vi "ISX3_Get_All_ISX3.vi"() -> (1 "A list of FT_Handel where an ISX-3 is connected to.\nThis handle must be used for further interaction \nwith the USB interface.":u32[](array[numeric]) format="%x")   [LabVIEW 2012, in "Sciospec ISX3 Impedance Analyzer.lvlib"]
uses:
  Sciospec ISX3 Impedance Analyzer.lvlib
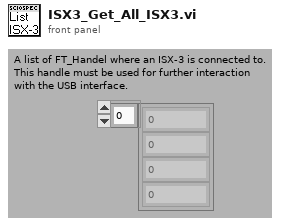
[diagram p1: front panel]
types:
  T1 = cluster{"Type":u32, "VID":string, "PID":string, "Serial Number":string, "Description":string}
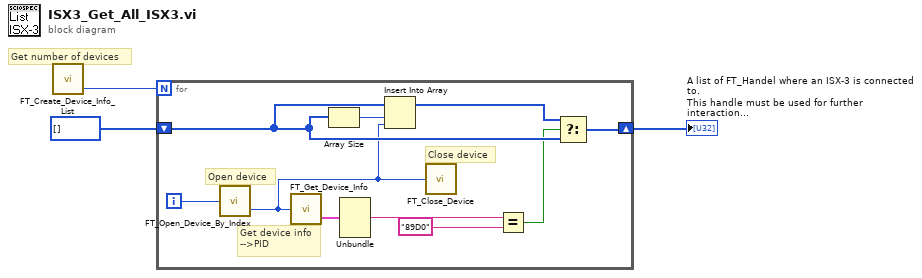
[diagram p0: block diagram]
diagram:
  # "Get number of devices"
  n1 = call "FT_Create_Device_Info_List.vi"() -> ("Number of Devices"=w1:u32)  [unwired: 1 out]
  n2 = for {
    N: w1 -> [_]
    shift-right: [w10] -> w2
    shift-left: u32[] [] -> [w11]
    i -> [w9]
    # "Close device"
    # "Get device info\n-->PID"
    # "Open device"
    n3 = call "FT_Open_Device_By_Index.vi"("Device Index"=w9) -> ("Handle"=w6:u32)  [unwired: 1 out]
    n4 = call "FT_Get_Device_Info.vi"("Handle"=w6) -> ("Device Information"=w8:T1)  [unwired: 1 out]
    n5 = Array Size(array=w11) -> (size(s)=w13:i32)
    n6 = Unbundle(w8) -> ("PID"=w4:string)  [unwired: 4 out]
    n7 = Insert Into Array(array=w11, index=w13, new element=w6) -> (w12:u32[])
    n8 = call "FT_Close_Device.vi"("Handle"=w6) -> ()  [unwired: 1 out]
    n9 = Equal?(x=w4, y="89D0") -> (x = y?=w5:bool)
    n10 = Select(t=w12, s=w5, f=w11) -> (s? t:f=w10:u32[])
  }
  "A list of FT_Handel where an ISX-3 is connected to.\nThis handle must be used for further interaction \nwith the USB interface." <- w2
